vi "Deinitialize Manifold.vi"(8 "error in (no error)":errorcluster, 11 "Gantry in":refnum<class "Gantry.lvclass">) -> (0 "error out":errorcluster, 3 "Gantry out":refnum<class "Gantry.lvclass">)   [LabVIEW 2022 SP3, in "Gantry.lvclass"]
uses:
  Gantry.lvclass
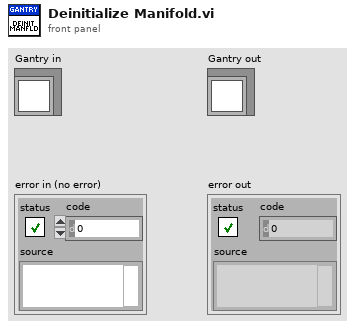
[diagram p1: front panel]
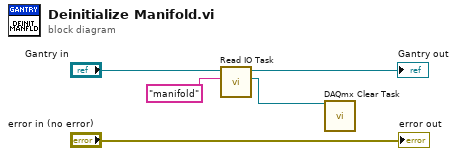
[diagram p0: block diagram]
diagram:
  n1 = call "Read IO Task.vi"("Task Name"="manifold", "Gantry in"="Gantry in") -> ("task/channels in"=w2:refnum<k21>, "Gantry out"=→"Gantry out":refnum<class "Gantry.lvclass">)  [unwired: 7 in, 1 out]
  n2 = call <vilib>:"DAQmx Clear Task.vi"("task in"=w2) -> ()  [unwired: 14 in, 1 out]
  "error out" <- "error in (no error)"
